vi "APC_9049_CA.vi"(6 "Window initi":u32, 7 "CAD/sample":dbl, 8 "MFB":dbl[](array[numeric])) -> (0 "CA97":dbl=0.43955275679402916, 1 "CA10CA90":dbl=0.43955275679402916, 2 "CA10":dbl=-8.49948440384458, 3 "CA50":dbl=0.43955275679402916, 4 "CA90":dbl=0.43955275679402916, 5 "CA03":dbl=-8.49948440384458)   [LabVIEW 2020]
panel:
  out "Window init [CAD]":dbl=-40.0
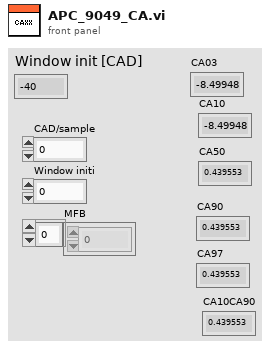
[diagram p1: front panel]
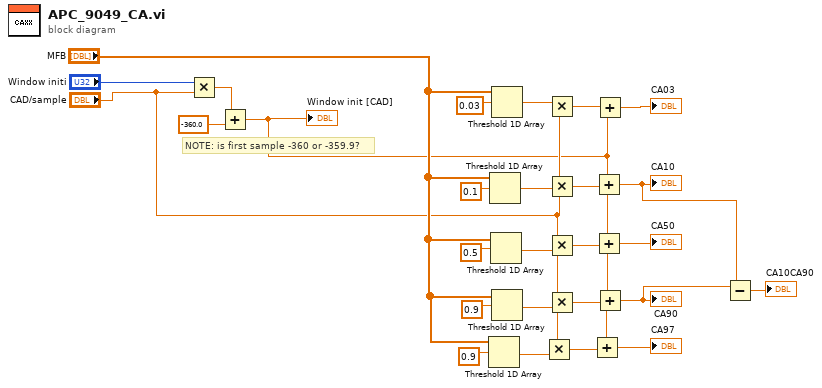
[diagram p0: block diagram]
diagram:
  # "NOTE: is first sample -360 or -359.9?"
  n1 = Multiply(x="Window initi", y="CAD/sample") -> (x*y=w24:dbl)
  n2 = Add(x=w24, y=-360.0) -> (x+y=w4:dbl)
  "Window init [CAD]" <- w4
  n3 = Threshold 1D Array(2:0.9 ("fractional index or x"), 3:"MFB") -> (0:w9:dbl)  [unwired: 1 in]
  n4 = Threshold 1D Array(2:0.1 ("fractional index or x"), 3:"MFB") -> (0:w23:dbl)  [unwired: 1 in]
  n5 = Threshold 1D Array(2:0.5 ("fractional index or x"), 3:"MFB") -> (0:w22:dbl)  [unwired: 1 in]
  n6 = Threshold 1D Array(2:0.03 ("fractional index or x"), 3:"MFB") -> (0:w13:dbl)  [unwired: 1 in]
  n7 = Threshold 1D Array(2:0.9 ("fractional index or x"), 3:"MFB") -> (0:w17:dbl)  [unwired: 1 in]
  n8 = Multiply(x="CAD/sample", y=w9) -> (x*y=w8:dbl)
  n9 = Multiply(x="CAD/sample", y=w13) -> (x*y=w12:dbl)
  n10 = Multiply(x="CAD/sample", y=w23) -> (x*y=w21:dbl)
  n11 = Multiply(x="CAD/sample", y=w22) -> (x*y=w20:dbl)
  n12 = Multiply(x="CAD/sample", y=w17) -> (x*y=w16:dbl)
  n13 = Add(x=w4, y=w8) -> (x+y=→"CA97":dbl)
  n14 = Add(x=w4, y=w21) -> (x+y=w2:dbl)
  "CA10" <- w2
  n15 = Add(x=w4, y=w20) -> (x+y=→"CA50":dbl)
  n16 = Add(x=w4, y=w12) -> (x+y=→"CA03":dbl)
  n17 = Add(x=w4, y=w16) -> (x+y=w3:dbl)
  "CA90" <- w3
  n18 = Subtract(x=w3, y=w2) -> (x-y=→"CA10CA90":dbl)
